vi "Init Series Graph.vi"(6 "Z Scale.Marker Values[]":cluster{"Numeric":dbl, "Numeric":u32}[](array[cluster]), 7 "Graphs":T1, 8 "error in (no error)":errorcluster, 9 "Shots":u32, 10 "Image Size":cluster{"Height":u32, "Width":u32}, 11 "Series Graph in":refnum<class "Series Graph.lvclass">) -> (0 "error out":errorcluster, 3 "Series Graph out":refnum<class "Series Graph.lvclass">)   [LabVIEW 2023, in "Series Graph.lvclass"]
uses:
  Series Graph.lvclass
  D:/git/Graph-Classes/Detail Graph/Detail Graph.lvclass
  Series Graph.lvclass/Series Graph.ctl
  Detail Graph/Detail Graph.lvclass
  D:/git/Graph-Classes/Base Graph/Base Graph.lvclass
  D:/git/Graph-Classes/Series Graph/Series Graph.lvclass
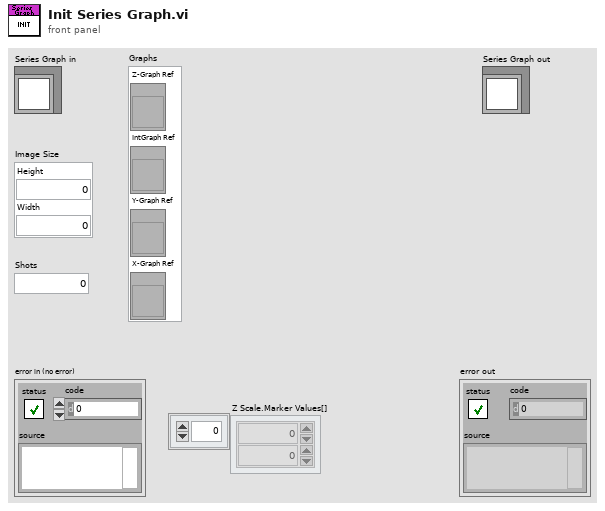
[diagram p1: front panel]
types:
  T1 = cluster{"Z-Graph Ref":refnum<vi>, "IntGraph Ref":refnum<vi>, "Y-Graph Ref":refnum<vi>, "X-Graph Ref":refnum<vi>}
  T2 = cluster{"IntGraph Ref":refnum<vi>, "Y-Graph Ref":refnum<vi>, "X-Graph Ref":refnum<vi>}
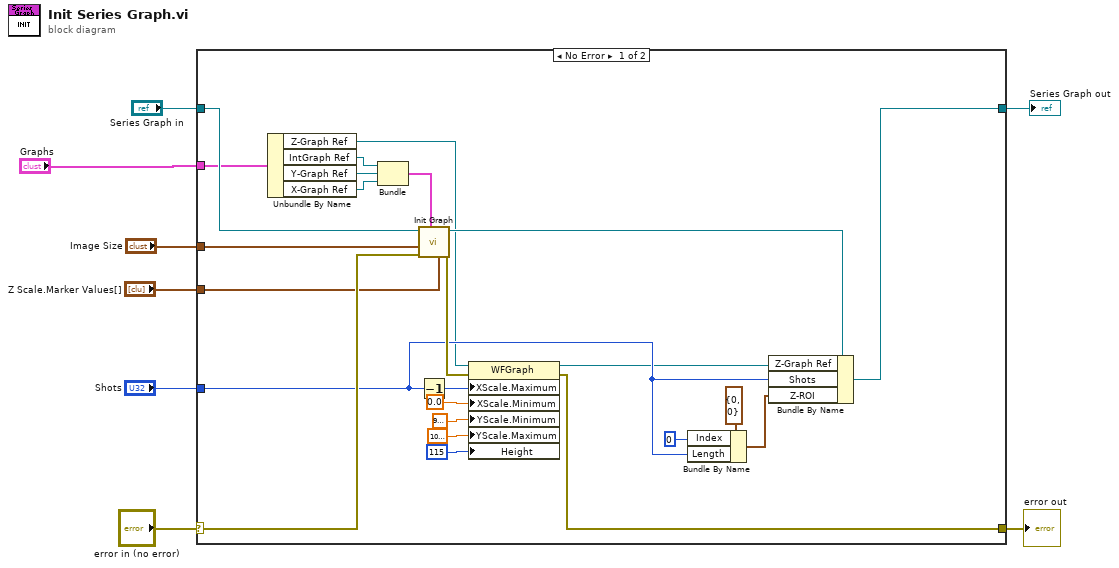
[diagram p0: block diagram]
diagram:
  n1 = case shown="No Error" "error in (no error)" {
    selector: "error in (no error)" -> [w32 w34]
    tunnel: [w10 w34] -> w7
    tunnel: [w25 w33] -> w2
    tunnel: "Series Graph in" -> [w31 w33]
    tunnel: "Image Size" -> [w18 _]
    tunnel: "Shots" -> [w23 _]
    tunnel: "Z Scale.Marker Values[]" -> [w30 _]
    tunnel: "Graphs" -> [w16 _]
    frame No Error {
      n2 = Unbundle By Name(w16) -> ("Z-Graph Ref"=w11:refnum<vi>, "IntGraph Ref"=w15:refnum<vi>, "Y-Graph Ref"=w14:refnum<vi>, "X-Graph Ref"=w13:refnum<vi>)
      n3 = Bundle("IntGraph Ref"=w15, "Y-Graph Ref"=w14, "X-Graph Ref"=w13) -> (w12:T2)  [unwired: 1 in]
      n4 = call "Init Graph.vi"("Z Scale.Marker Values[]"=w30, "Graphs"=w12, "error in (no error)"=w32, "Images Size"=w18, "Detail Graph.lvclass"=w31) -> ("error out"=w24:errorcluster, "Detail Graph out.lvclass"=w26:refnum<class "Series Graph.lvclass">)  [unwired: 5 in]
      n5 = Decrement(x=w23) -> (x-1=w17:u32)
      n6 = property class="WFGraph"(reference=w11, error in=w24, "XScale.Maximum"=w17, "XScale.Minimum"=0.0 ("X Scale.Range:Minimum"), "YScale.Minimum"=9000.0 ("Y Scale.Range:Minimum"), "YScale.Maximum"=10000.0 ("Y Scale.Range:Maximum"), "Height"=u32 115 ("Plot Area:Size:Height")) -> (reference out=w9:refnum<vi>, error out=w10:errorcluster)
      n7 = Bundle By Name(cluster=cluster{"Index":u32, "Length":u32} {"Index"=0, "Length"=0} ("Z-ROI"), "Index"=u32 0, "Length"=w23) -> (w27:cluster{"Index":u32, "Length":u32})
      n8 = Bundle By Name(cluster=w26, "Z-Graph Ref"=w9, "Shots"=w23, "Z-ROI"=w27) -> (w25:refnum<class "Series Graph.lvclass">)
    }
    frame Error {
    }
  }
  "error out" <- w7
  "Series Graph out" <- w2
